vi "Test5.vi"(9 "TorF":bool, 11 "Data In":T1) -> (3 "Data Out":T1)   [LabVIEW 2014]
uses:
  controls/Data.ctl
panel:
  # "日期"
  # "機種名稱"
  # "機種代號"
  # "商品條碼"
  # "台"
  # "OK"
  # "NG"
  # "台"
  # "總計"
  # "台"
  # "日期"
  # "機種名稱"
  # "機種代號"
  # "商品條碼"
  # "台"
  # "OK"
  # "NG"
  # "台"
  # "總計"
  # "台"
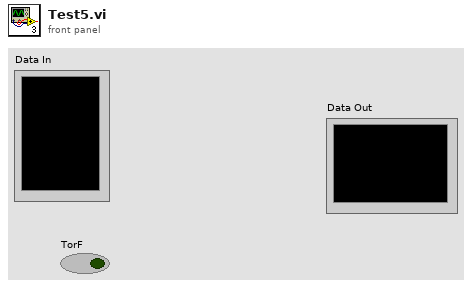
[diagram p1: front panel]
types:
  T1 = typedef "Data.ctl" = cluster{"Date":string, "BarCode1":string, "BarCode2":string, "BarCode3":string, "Message":string, "OK Count":u16, "NG Count":u16, "Total Count":u16, "ModelData":string[][], "OK&NG":bool, "COM1":refnum<visa-resource-name>, "COM2":refnum<visa-resource-name>, "IO":i32, "Time":u32, "TCP":refnum<k5>, "TCP 2":refnum<k5>}
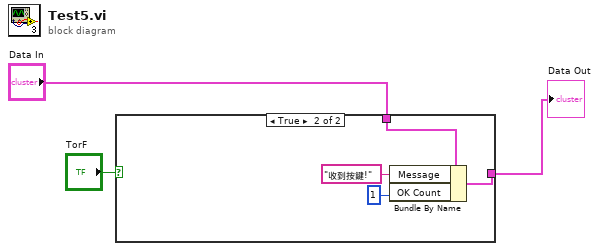
[diagram p0: block diagram]
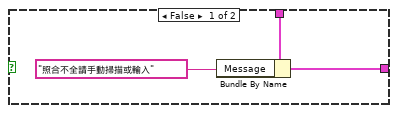
[diagram p2: hidden frame]
diagram:
  n1 = case shown="True" "TorF" {
    tunnel: "Data In" -> [w5 w10]
    tunnel: [w4 w9] -> w1
    frame False {
      n2 = Bundle By Name(cluster=w5, "Message"="照合不全請手動掃描或輸入" ("string")) -> (w4:T1)
    }
    frame True {
      n3 = Bundle By Name(cluster=w10, "Message"="收到按鍵!", "OK Count"=u16 1) -> (w9:T1)
    }
  }
  "Data Out" <- w1
